vi "Write Reset.vi"(8 "error in (no error)":errorcluster, 10 "Reset":bool, 11 "DAQ Class in":refnum<class "DAQ Class.lvclass">) -> (0 "error out":errorcluster, 3 "DAQ Class out":refnum<class "DAQ Class.lvclass">)   [LabVIEW 2014, in "DAQ Class.lvclass"]
uses:
  DAQ Class.lvclass
  DAQ Class.lvclass/DAQ Class.ctl
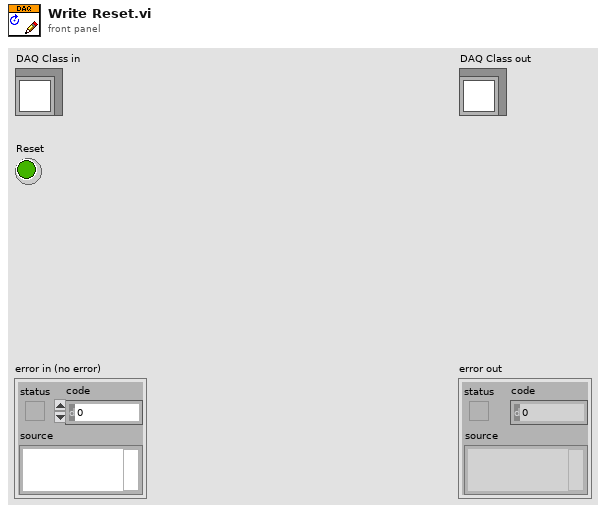
[diagram p1: front panel]
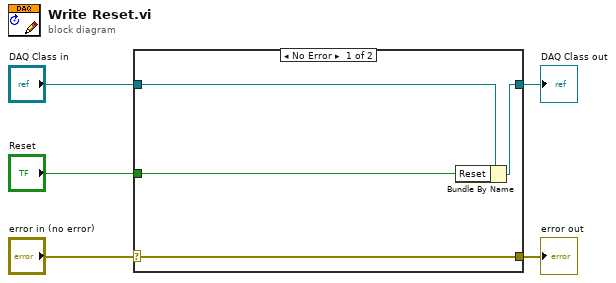
[diagram p0: block diagram]
diagram:
  n1 = case shown="No Error" "error in (no error)" {
    selector: "error in (no error)" -> [w9 w10]
    tunnel: [w9 w10] -> w4
    tunnel: [w7 w11] -> w2
    tunnel: "DAQ Class in" -> [w8 w11]
    tunnel: "Reset" -> [w6 _]
    frame No Error {
      n2 = Bundle By Name(cluster=w8, "Reset"=w6) -> (w7:refnum<class "DAQ Class.lvclass">)
    }
    frame Error {
    }
  }
  "error out" <- w4
  "DAQ Class out" <- w2
